vi "Open and Configure Device Core.vi"(0 "USRP RIO Device":T2, 5 "reference frequency source":string(combo)="Internal", 7 "which bitfile":string(combo)="Time", 9 "wait for gps lock?":bool, 11 "error in":errorcluster, 12 "rx config":T4={"channel configuration"=[], "transfer mode"=enum."Finite", "sample rate"=10000000.0, "number of samples"=8192, "start trigger"=enum."Immediate"} {"channel configuration"."channel configuration"."frequency" format="%#.3pHz"; "channel configuration"."channel configuration"."lo frequency" format="%#.3pHz"; "channel configuration"."channel configuration"."level" format="%#_gdBm"; "sample rate" format="%#.3pS/s"}, 13 "tx config":T5={"channel configuration"=[], "transfer mode"=enum."Finite", "sample rate"=10000000.0, "number of samples"=8192, "start trigger"=enum."Immediate", "tone frequency"=100000.0} {"channel configuration"."channel configuration"."frequency" format="%#.3pHz"; "channel configuration"."channel configuration"."lo frequency" format="%#.3pHz"; "channel configuration"."channel configuration"."level" format="%#_gdBm"; "tone frequency" format="%#.3pHz"; "sample rate" format="%#.3pS/s"}, 14 "lo config":T1) -> (2 "rx channels":T7={"rx config"={"channel configuration"=[], "transfer mode"=enum."Finite", "sample rate"=10000000.0, "number of samples"=8192, "start trigger"=enum."Immediate"}, "reference frequency source"="Internal", "rx.data sink"=enum."Host", "rx.enabled channels"=[], "vertical range"=[], "rx.coerced configurations"={"coerced frequencies"=[], "coerced lo frequencies"=[], "coerced levels"=[], "coerced sample rates"=[]}} {"rx.coerced configurations"."coerced sample rates" format="%#.3pS/s"; "rx.coerced configurations"."coerced levels" format="%#.3gdBm"; "rx.coerced configurations"."coerced lo frequencies" format="%#.3pHz"; "rx.coerced configurations"."coerced frequencies" format="%#.3pHz"; "rx config"."channel configuration"."channel configuration"."frequency" format="%#.3pHz"; "rx config"."channel configuration"."channel configuration"."lo frequency" format="%#.3pHz"; "rx config"."channel configuration"."channel configuration"."level" format="%#_gdBm"; "rx config"."sample rate" format="%#.3pS/s"; "vertical range" format="%#.3pVpp"}, 3 "tx channels":T6={"tx config"={"channel configuration"=[], "transfer mode"=enum."Finite", "sample rate"=10000000.0, "number of samples"=8192, "start trigger"=enum."Immediate", "tone frequency"=100000.0}, "reference frequency source"="Internal", "tx.data source"=enum."Host", "tx.enabled channels"=[], "I"=[], "Q"=[], "tx.coerced configurations"={"coerced frequencies"=[], "coerced lo frequencies"=[], "coerced levels"=[], "coerced sample rates"=[]}} {"tx.coerced configurations"."coerced sample rates" format="%#.3pS/s"; "tx.coerced configurations"."coerced levels" format="%#.3gdBm"; "tx.coerced configurations"."coerced lo frequencies" format="%#.3pHz"; "tx.coerced configurations"."coerced frequencies" format="%#.3pHz"; "tx config"."channel configuration"."channel configuration"."frequency" format="%#.3pHz"; "tx config"."channel configuration"."channel configuration"."lo frequency" format="%#.3pHz"; "tx config"."channel configuration"."channel configuration"."level" format="%#_gdBm"; "tx config"."tone frequency" format="%#.3pHz"; "tx config"."sample rate" format="%#.3pS/s"}, 4 "niUsrpRio Session (out)":T9 {"Daughterboard Clock Rate" format="%#.3pHz"; "FPGA Data Clock Rate" format="%#.3pHz"; "Data Clock Rate" format="%#.3pHz"; "Characterization Data"."Frequencies [Hz]" format="%#_6p"; "EEPROM Characterization Header"."Pointer to Device Data Header" format="%x"; "EEPROM Characterization Header"."Checksum" format="%x"; "Device Data Header"."Pointer to Characterization Data" format="%x"; "Device Data Header"."Checksum" format="%x"; "EEPROM Header"."Pointer to User Header" format="%x"; "EEPROM Header"."Pointer to Factory Header" format="%x"; "EEPROM Header"."Product Code" format="%x"; "EEPROM Header"."Checksum" format="%x"}, 6 "rx.coerced configurations":T8 {"coerced sample rates" format="%#.3pS/s"; "coerced levels" format="%#.3gdBm"; "coerced lo frequencies" format="%#.3pHz"; "coerced frequencies" format="%#.3pHz"}, 8 "tx.coerced configurations":T8 {"coerced sample rates" format="%#.3pS/s"; "coerced levels" format="%#.3gdBm"; "coerced lo frequencies" format="%#.3pHz"; "coerced frequencies" format="%#.3pHz"}, 10 "tx.output waveform":waveform(dbl)[](graph), 15 "error out":errorcluster)   [LabVIEW 2021]
uses:
  <instrlib>/niUsrpRio/Config/v1/Host/Public/niUsrpRio Session.ctl
  <instrlib>/_niInstr/Register Bus/v0/Host/Public/Register Bus Session.ctl
  <instrlib>/_niInstr/Register Bus/v0/Host/Private/Session Data.ctl
  <instrlib>/niUsrpRio/Config/v1/Host/Private/DB Queue Reference.ctl
  <instrlib>/niUsrpRio/Config/v1/Host/Private/Daughterboard Data.ctl
  <instrlib>/niUsrpRio/Config/v1/Host/Private/ATR state data.ctl
  <instrlib>/niUsrpRio/Config/v1/Host/Private/Antenna Configuration.ctl
  <instrlib>/niUsrpRio/Config/v1/Host/Private/CPLD Power Mode.ctl
  <instrlib>/niUsrpRio/Config/v1/Host/Public/EEPROM Header.ctl
  <instrlib>/niUsrpRio/Config/v1/Host/Public/EEPROM Device Data Header.ctl
  <instrlib>/niUsrpRio/Config/v1/Host/Public/EEPROM Characterization Header.ctl
  <instrlib>/niUsrpRio/Config/v1/Host/Public/Characterization Data.ctl
  <instrlib>/niUsrpRio/Config/v1/Host/Public/IQ Imbalance.ctl
  Rx Channels.ctl
  Start Trigger.ctl
  Tx Channels.ctl
  <vilib>/userdefined/Silver/nirio_resource_slv.ctl
  <instrlib>/_niInstr/Register Bus/v0/Host/niInstr Register Bus v0 Host.lvlib
  <instrlib>/niUsrpRio/Config/v1/Host/niUsrpRio Config v1 Host.lvlib
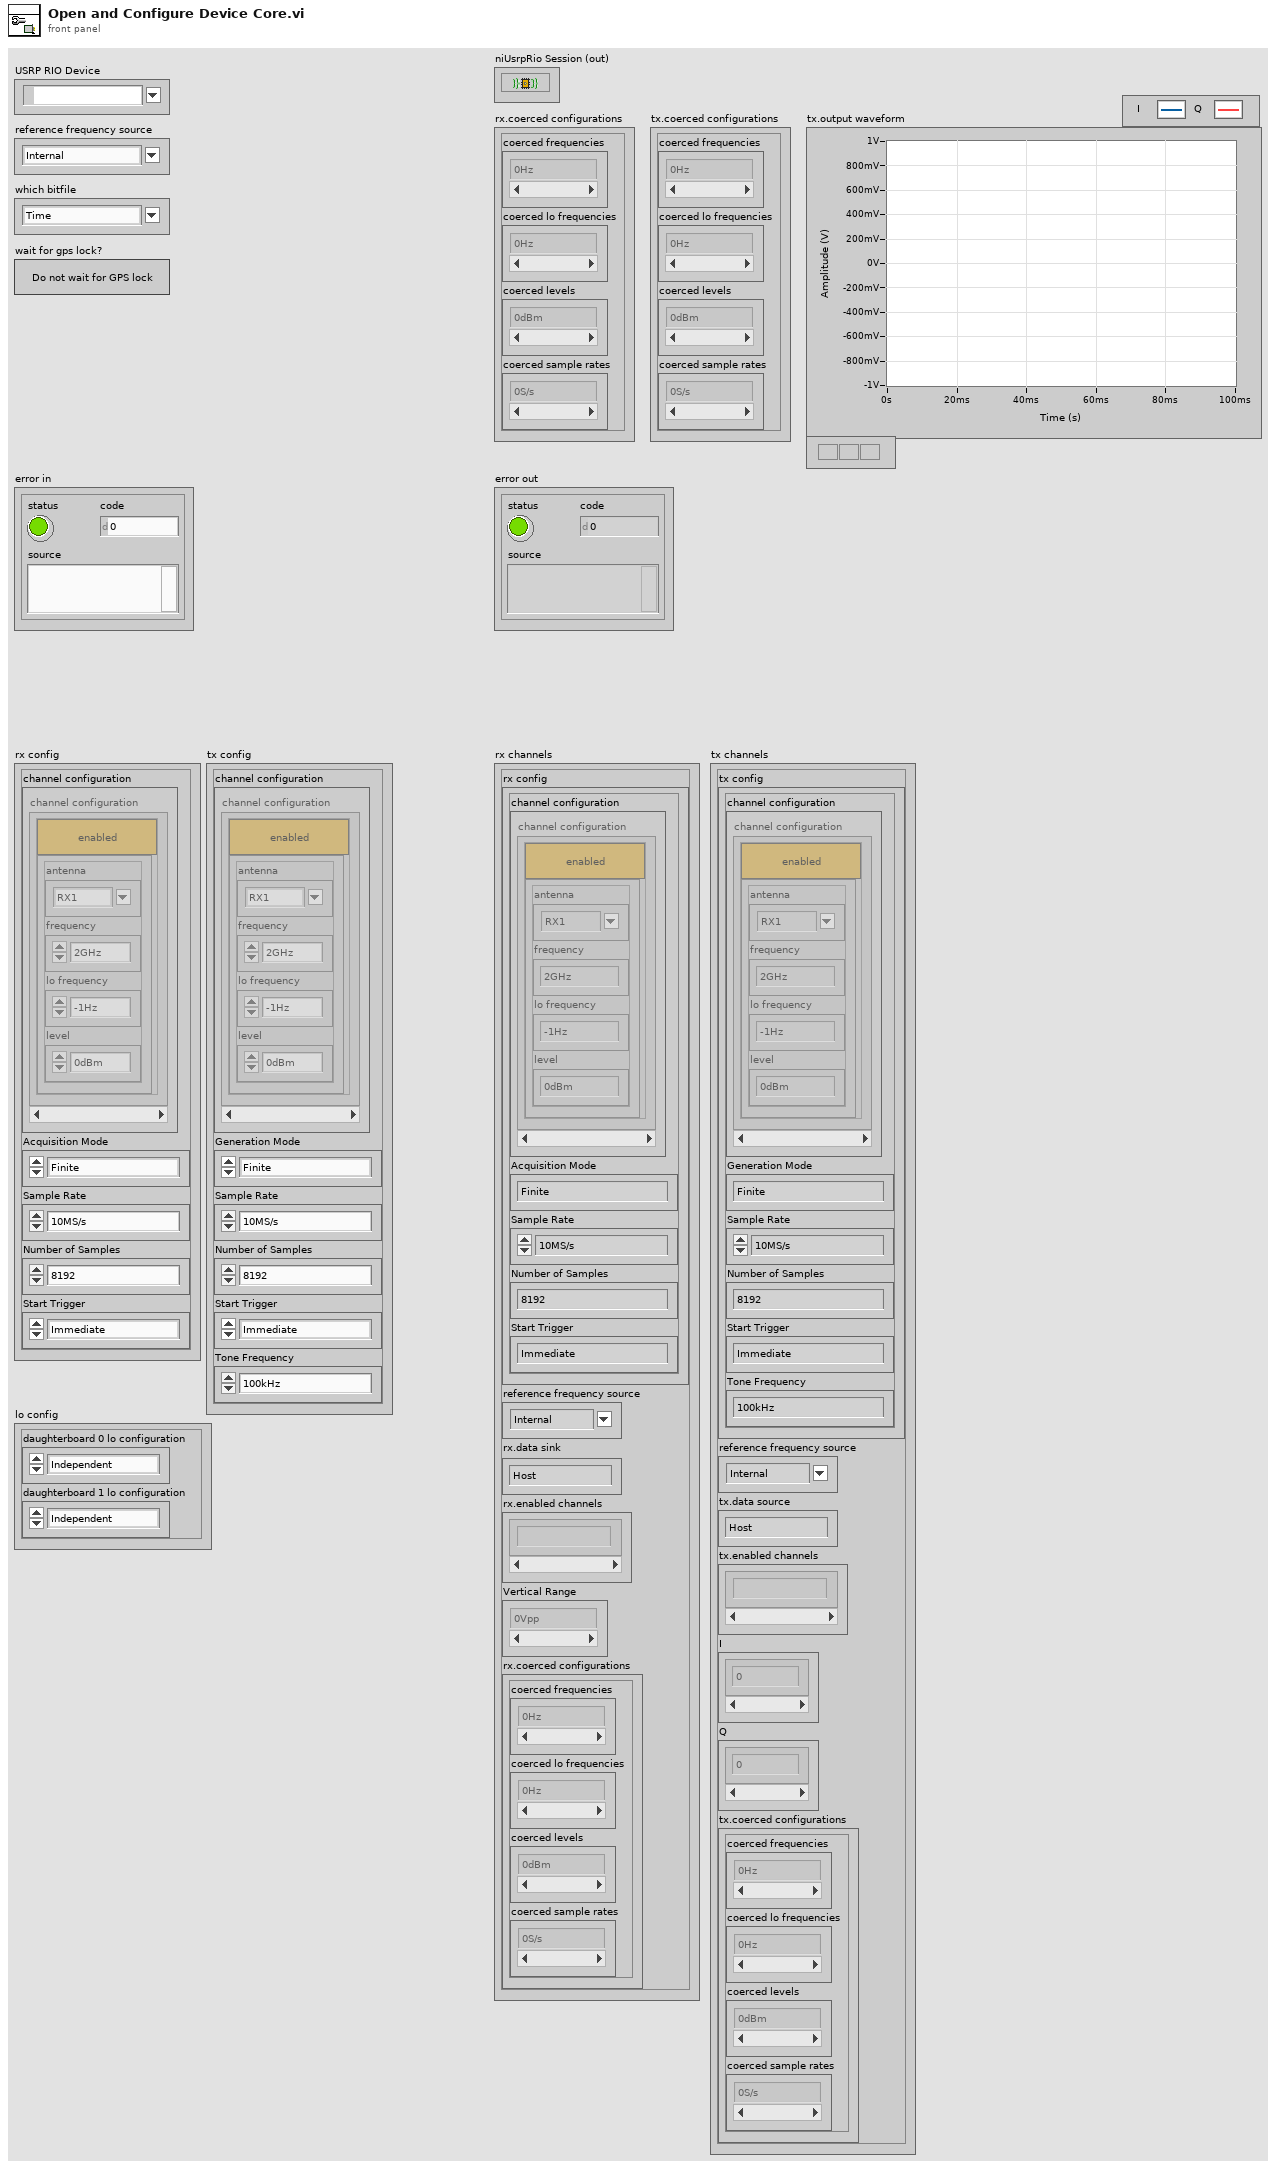
[diagram p1: front panel]
types:
  T1 = cluster{"daughterboard 0 lo configuration":enum16{"Independent", "Import", "Shared and Export", "Reimport", "Shared"}, "daughterboard 1 lo configuration":enum16{"Independent", "Import", "Shared and Export", "Reimport", "Shared"}}
  T2 = typedef "nirio_resource_slv.ctl" = tag
  T3 = typedef "Start Trigger.ctl" = enum8{"Software", "Digital Edge", "Rx Start Trigger", "Tx Start Trigger", "Immediate", "Future Time Event"}
  T4 = cluster{"channel configuration":cluster{"channel enable":bool, "channel configuration":cluster{"antenna":string, "frequency":dbl, "lo frequency":dbl, "level":dbl}}[], "transfer mode":enum16{"Finite", "Continuous"}, "sample rate":dbl, "number of samples":u32, "start trigger":T3}
  T5 = cluster{"channel configuration":cluster{"channel enable":bool, "channel configuration":cluster{"antenna":string, "frequency":dbl, "lo frequency":dbl, "level":dbl}}[], "transfer mode":enum16{"Finite", "Continuous"}, "sample rate":dbl, "number of samples":u32, "start trigger":T3, "tone frequency":dbl}
  T6 = typedef "Tx Channels.ctl" = cluster{"tx config":cluster{"channel configuration":cluster{"channel enable":bool, "channel configuration":cluster{"antenna":string, "frequency":dbl, "lo frequency":dbl, "level":dbl}}[], "transfer mode":enum16{"Finite", "Continuous"}, "sample rate":dbl, "number of samples":u32, "start trigger":T3, "tone frequency":dbl}, "reference frequency source":string, "tx.data source":enum16{"SFP Port 0", "SFP Port 1", "Host"}, "tx.enabled channels":string[], "I":i16[], "Q":i16[], "tx.coerced configurations":cluster{"coerced frequencies":dbl[], "coerced lo frequencies":dbl[], "coerced levels":dbl[], "coerced sample rates":dbl[]}}
  T7 = typedef "Rx Channels.ctl" = cluster{"rx config":cluster{"channel configuration":cluster{"channel enable":bool, "channel configuration":cluster{"antenna":string, "frequency":dbl, "lo frequency":dbl, "level":dbl}}[], "transfer mode":enum16{"Finite", "Continuous"}, "sample rate":dbl, "number of samples":u32, "start trigger":T3}, "reference frequency source":string, "rx.data sink":enum16{"SFP Port 0", "SFP Port 1", "Host"}, "rx.enabled channels":string[], "vertical range":dbl[], "rx.coerced configurations":cluster{"coerced frequencies":dbl[], "coerced lo frequencies":dbl[], "coerced levels":dbl[], "coerced sample rates":dbl[]}}
  T8 = cluster{"coerced frequencies":dbl[], "coerced lo frequencies":dbl[], "coerced levels":dbl[], "coerced sample rates":dbl[]}
  T9 = typedef "niUsrpRio Config v1 Host.lvlib/niUsrpRio Session.ctl" = cluster{"FPGA Interface":refnum<k20>, "RIO Interface Number":u32, "Data Clock Rate":u32, "FPGA Data Clock Rate":u32, "Global Settings Register Bus":T10, "Radio 0 Settings Register Bus":T10, "Radio 1 Settings Register Bus":T10, "Radio Settings Bus Semaphore":T11, "DB Queues":T12[], "Characterization Data Valid?":bool, "EEPROM Header":T13, "Device Data Header":T14, "EEPROM Characterization Header":T15, "Characterization Data":T16[], "FPGA Current Version":u32, "FPGA Oldest Compatible Version":u32, "Fixed Logic Current Version":u32, "Fixed Logic Oldest Compatible Version":u32, "FPGA Radio Settings Bus Current Version":u32, "FPGA Radio Settings Bus Oldest Compatible Version":u32, "FPGA Board Config Current Version":u32, "FPGA Board Config Oldest Compatible Version":u32, "Daughterboard Clock Rate":u32, "daughterboard configuration session handles":u64[]}
  T10 = typedef "niInstr Register Bus v0 Host.lvlib/Register Bus Session.ctl" = refnum<queue>
  T11 = typedef "Semaphore RefNum" = refnum<k1>
  T12 = typedef "niUsrpRio Config v1 Host.lvlib/DB Queue Reference.ctl" = refnum<queue>
  T13 = typedef "niUsrpRio Config v1 Host.lvlib/EEPROM Header.ctl" = cluster{"Checksum":u32, "Product Code":u16, "Hardware Current Version":u16, "Hardware Oldest Compatible Version":u16, "EEPROM Map Current Version":u16, "EEPROM Map Oldest Compatible Version":u16, "User Password":string, "Pointer to Factory Header":u32, "Pointer to User Header":u32, "Recommended Interval":u16, "Number of Reserved Bytes":i32, "Number of Daughterboards":u8, "Daughterboard IDs":u16[], "Daughterboard Serial Numbers":string[]}
  T14 = typedef "niUsrpRio Config v1 Host.lvlib/EEPROM Device Data Header.ctl" = cluster{"Checksum":u32, "Number of Channels":u8, "Number of Gain Settings":u16[], "Pointer to Characterization Data":u32[], "Number of Reserved Bytes":i32, "Number of Frequencies":u16[]}
  T15 = typedef "niUsrpRio Config v1 Host.lvlib/EEPROM Characterization Header.ctl" = cluster{"Checksum":u32, "Date":timestamp, "Temperature":sgl, "Misc. Info":string, "Pointer to Device Data Header":u32, "Number of Reserved Bytes":i32}
  T16 = typedef "niUsrpRio Config v1 Host.lvlib/Characterization Data.ctl" = cluster{"Gains[dB]":dbl[], "Frequencies [Hz]":dbl[], "IQ Imbalance Table":T17[], "Measured Gains[dB]":dbl[][]}
  T17 = typedef "niUsrpRio Config v1 Host.lvlib/IQ Imbalance.ctl" = cluster{"Gain Imbalance [linear]":dbl, "Phase Imbalance [radians]":dbl, "Offset":cdb}
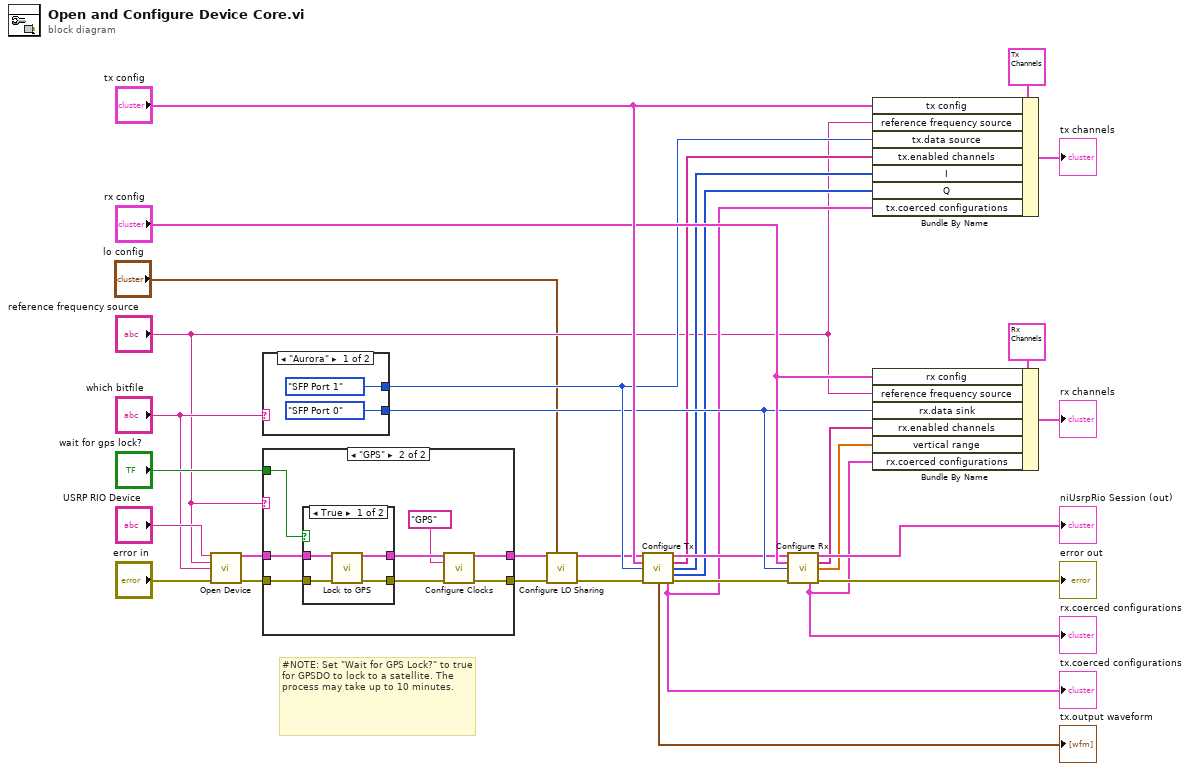
[diagram p0: block diagram]
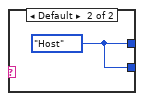
[diagram p2: hidden frame]
diagram:
  # "#NOTE: Set \"Wait for GPS Lock?\" to true for GPSDO to lock to a satellite. The process may take up to 10 minutes."
  n1 = call "Open Device.vi"("USRP RIO device"="USRP RIO Device", "Reference Frequency Source"="reference frequency source", "which bitfile"="which bitfile", "error in"="error in") -> ("niUsrpRio Session (out)"=w11:T9, "error out"=w10:errorcluster)  [unwired: 10 in]
  n2 = case shown="\"Aurora\"" "which bitfile" {
    tunnel: [enum16{"SFP Port 0", "SFP Port 1", "Host"}."SFP Port 1" ("data stream config") w35] -> w28
    tunnel: [enum16{"SFP Port 0", "SFP Port 1", "Host"}."SFP Port 0" ("data stream config") w35] -> w27
    frame "Aurora" {
    }
    frame Default {
      w35 = enum16{"SFP Port 0", "SFP Port 1", "Host"}."Host" ("data stream config")
    }
  }
  n3 = case shown="\"GPS\"" "reference frequency source" {
    tunnel: w11 -> [w37 w45]
    tunnel: [w37 w40] -> w4
    tunnel: [w36 w42] -> w3
    tunnel: w10 -> [w36 w44]
    tunnel: "wait for gps lock?" -> [_ w38]
    frame Default {
    }
    frame "GPS" {
      n4 = case shown="True" w38 {
        tunnel: w45 -> [w47 w51]
        tunnel: [w49 w51] -> w41
        tunnel: [w48 w50] -> w43
        tunnel: w44 -> [w46 w50]
        frame True {
          n5 = call "Lock to GPS.vi"("niUsrpRio Session"=w47, "error in"=w46) -> ("niUsrpRio Session (out)"=w49:T9, "error out"=w48:errorcluster)  [unwired: 12 in]
        }
        frame False {
        }
      }
      n6 = call "Configure Clocks.vi"("niUsrpRio Session"=w41, "Reference Frequency Source"="GPS", "error in"=w43) -> ("niUsrpRio Session (out)"=w40:T9, "error out"=w42:errorcluster)  [unwired: 11 in]
    }
  }
  n7 = call "Configure LO Sharing.vi"("niUsrpRio Session in"=w4, "lo config"="lo config", "error in"=w3) -> ("niUsrpRio Session out"=w5:T9, "error out"=w2:errorcluster)  [unwired: 11 in]
  n8 = call "Configure Tx.vi"("niUsrpRio Session"=w5, "tx config"="tx config", "tx.data source"=w28, "error in"=w2) -> ("niUsrpRio Session (out)"=w19:T9, "tx.enabled channels"=w15:string[], "I"=w16:i16[], "Q"=w17:i16[], "tx.output waveform"=→"tx.output waveform":waveform(dbl)[], "tx.coerced configurations"=w18:T8, "error out"=w20:errorcluster)  [unwired: 5 in]
  "tx.coerced configurations" <- w18
  n9 = call "Configure Rx.vi"("niUsrpRio Session"=w19, "rx config"="rx config", "rx.data sink"=w27, "error in"=w20) -> ("niUsrpRio Session (out)"=→"niUsrpRio Session (out)":T9, "rx.enabled channels"=w24:string[], "vertical range"=w23:dbl[], "rx.coerced configurations"=w21:T8, "error out"=→"error out":errorcluster)  [unwired: 7 in]
  "rx.coerced configurations" <- w21
  n10 = Bundle By Name(cluster=T6 {"tx config"={"channel configuration"=[], "transfer mode"=enum."Finite", "sample rate"=10000000.0, "number of samples"=8192, "start trigger"=enum."Immediate", "tone frequency"=100000.0}, "reference frequency source"="Internal", "tx.data source"=enum."Host", "tx.enabled channels"=[], "I"=[], "Q"=[], "tx.coerced configurations"={"coerced frequencies"=[], "coerced lo frequencies"=[], "coerced levels"=[], "coerced sample rates"=[]}} ("tx channels"), "tx config"="tx config", "reference frequency source"="reference frequency source", "tx.data source"=w28, "tx.enabled channels"=w15, "I"=w16, "Q"=w17, "tx.coerced configurations"=w18) -> (→"tx channels":T6)
  n11 = Bundle By Name(cluster=T7 {"rx config"={"channel configuration"=[], "transfer mode"=enum."Finite", "sample rate"=10000000.0, "number of samples"=8192, "start trigger"=enum."Immediate"}, "reference frequency source"="Internal", "rx.data sink"=enum."Host", "rx.enabled channels"=[], "vertical range"=[], "rx.coerced configurations"={"coerced frequencies"=[], "coerced lo frequencies"=[], "coerced levels"=[], "coerced sample rates"=[]}} ("rx channels"), "rx config"="rx config", "reference frequency source"="reference frequency source", "rx.data sink"=w27, "rx.enabled channels"=w24, "vertical range"=w23, "rx.coerced configurations"=w21) -> (→"rx channels":T7)
